vi "VerticalTrajectory.vi"(2 "speed 2":i32, 3 "speed 1":i32, 4 "step":dbl, 5 "z2":dbl, 6 "z1":dbl, 7 "x":dbl) -> ()   [LabVIEW 2018]
panel:
  out "q1":dbl
  out "q2":dbl
  in  "dt":dbl
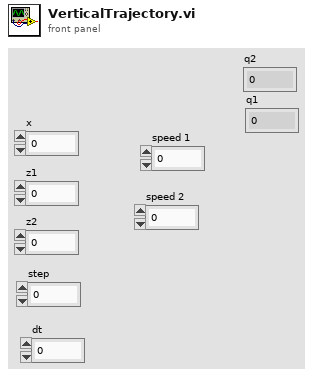
[diagram p1: front panel]
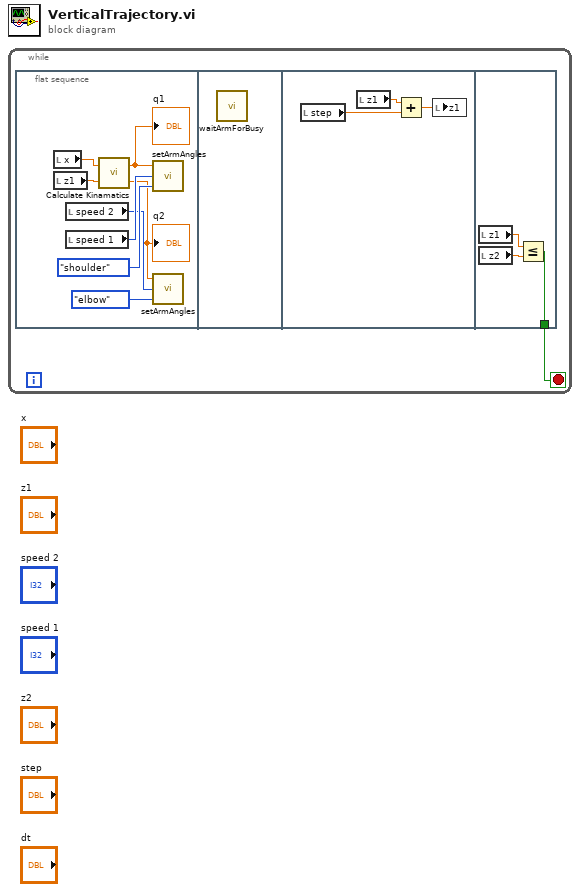
[diagram p0: block diagram]
diagram:
  n1 = while {
    stop <- w1 stop-if-true
    n2 = flat-sequence {
      tunnel: [w13] -> w1
      frame #0 {
        n3 = local read "x"() -> (w9:dbl)
        n4 = local read "z1"() -> (w8:dbl)
        n5 = local read "speed 2"() -> (w2:i32)
        n6 = local read "speed 1"() -> (w5:i32)
        n7 = call "Calculate Kinamatics.vi"("y"=w8, "x"=w9) -> ("q2"=w3:dbl, "q1"=w4:dbl)
        "q2" <- w3
        "q1" <- w4
        n8 = call "setArmAngles.vi"("Enum"=enum16{"shoulder", "elbow", "wrist"}."shoulder", "speed"=w5, "angle"=w4) -> ()  [unwired: 1 in]
        n9 = call "setArmAngles.vi"("Enum"=enum16{"shoulder", "elbow", "wrist"}."elbow", "speed"=w2, "angle"=w3) -> ()  [unwired: 1 in]
      }
      frame #1 {
        n10 = call "waitArmForBusy.vi"() -> ()  [unwired: 12 in]
      }
      frame #2 {
        n11 = local read "step"() -> (w11:dbl)
        n12 = local read "z1"() -> (w12:dbl)
        n13 = Add(x=w12, y=w11) -> (x+y=w10:dbl)
        n14 = local write "z1"(w10) -> ()
      }
      frame #3 {
        n15 = local read "z1"() -> (w14:dbl)
        n16 = local read "z2"() -> (w15:dbl)
        n17 = Less Or Equal?(x=w14, y=w15) -> (x <= y?=w13:bool)
      }
    }
  }
